vi "Tigella_Main.vi"() -> ()   [LabVIEW 2024]
uses:
  PS3 Control V8.6/Controls/PS3 Controls.ctl
  <vilib>/Instr/_visa.llb/VISA Set IO Buffer Mask.ctl
  <vilib>/Instr/_visa.llb/VISA Configure Serial Port (Instr).vi
panel:
  out "MOF_Motor2":u8=3
  out "MOF_Motor1":u8=2
  out "read buffer":string
  out "return count":u32
  in  "VISA resource name out":refnum<visa-resource-name>
  in  "parity (0:none)":enum16{"None", "Odd", "Even", "Mark", "Space"}(ring)
  in  "data bits (8)":u16=8 min=5 max=8 step=1
  in  "baud rate (9600)":u32=115200
  out "M2_I_Adsorbed":i64
  out "M1_I_Adsorbed":i64
  out "Warning_M2":bool=TRUE
  out "Warning_M1":bool=TRUE
  out "Error_M2":bool=TRUE
  out "Error_M1":bool=TRUE
  out "STM _WIFIConnected":bool
  in  "Tab Control":T1(tab)
  out "Listbox_Motors_errors":i32(listbox)
  in  "Homing_M1":bool
  in  "velocity_profileM1":bool
  in  "position_profile_M1":bool
  out "Actual_Modality_M1":string
  in  "Start_Remote_Node_M1":bool
  in  "Stop_Remote_Node_M1":bool
  in  "Reset_Node_M1":bool
  in  "Reset_Communication_M1":bool
  in  "Enter_Pre_Operational_M1":bool
  out "NMT_State_M1":string
  in  "Shutdown_M1":bool
  out "Driver_State_M1":string
  in  "Disable_voltage_M1":bool
  in  "Switch_On_M1":bool
  in  "Disable_operation_M1":bool
  in  "Enable_Operation_M1":bool
  in  "Fault_Reset_M1":bool
  in  "Quick_Stop_M1":bool
  in  "Quick_Stop_M2":bool
  in  "Fault_Reset_M2":bool
  in  "Enable_Operation_M2":bool
  in  "Disable_operation_M2":bool
  in  "Switch_On_M2":bool
  in  "Disable_voltage_M2":bool
  out "Driver_State_M2":string
  in  "Shutdown_M2":bool
  out "NMT_State_M2":string
  in  "Enter_Pre_Operational_M2":bool
  in  "Reset_Communication_M2":bool
  in  "Reset_Node_M2":bool
  in  "Stop_Remote_Node_M2":bool
  in  "Start_Remote_Node_M2":bool
  out "Actual_Modality_M2":string
  in  "position_profile_M2":bool
  in  "velocity_profileM2":bool
  in  "Homing_M2":bool
  out "Listbox_Motors_errors 2":i32(listbox)
  in  "Halt_M2":bool
  out "M2_Velocity":i64
  out "M2_Position":i64
  in  "Change_set_immediately_M2":bool=TRUE
  in  "ABS/REL_M2":bool=TRUE
  in  "Target_Position_M2":i32
  in  "Target_speed_M2":i32
  in  "GO_TO_M2":bool
  out "M2_Following/homing error":bool=TRUE
  out "M2_Setpoint acknowledge/Homing attained":bool=TRUE
  out "M2_target_reached":bool=TRUE
  out "Saved_position_negative_M2":i64
  out "Saved_position_positive_M2":i64
  out "Motor2_FULL_Operational":bool=TRUE
  in  "Halt_M1":bool
  out "End-Stop_sensor":bool=TRUE
  out "Homing_Sensor":bool=TRUE
  out "M1_Velocity":i64
  out "M1_Position":i64
  in  "Change_set_immediately_M1":bool=TRUE
  in  "ABS/REL_M1":bool=TRUE
  in  "Target_Position_M1":i32
  in  "Target_speed_M1":i32
  in  "GO_TO_M1":bool
  out "M1_Following/homing error":bool=TRUE
  out "M1_Setpoint acknowledge/Homing attained":bool=TRUE
  out "M1_Internal_limit_\nactive":bool=TRUE
  out "M1_target_reached":bool=TRUE
  out "Saved_position_negative_M1":i64
  out "Saved_position_positive_M1":i64
  out "Motor1_FULL_Operational":bool=TRUE
  in  "Open_CAM":bool
  out "Controller_ERROR_STATUS":errorcluster
  out "PS3/4_controller_status":bool
  in  "Connect_PS3/4_controller":bool
  out "PS3 Controls":T2 {"Left Analogue Stick X" scale=-32768.0..32768.0; "Left Analogue Stick Y" scale=32768.0..-32768.0; "Right Analogue Stick X" scale=-32768.0..32768.0; "Right Analogue Stick Y" scale=32768.0..-32768.0; "X Rotation" scale=-32768.0..32768.0; "Y Rotation" scale=-32768.0..32768.0; "L2 Pressure" scale=0.0..32768.0; "Numeric" format="%d°"}
  in  "ID_Motor2":u8=3
  in  "ID_Motor1":u8=2
  out "Position_traction":i64
  out "Position_steering":i64
  out "Velocity_Traction":i64
  out "Velocity_steering":i64
  in  "SET_nodes":bool
  in  "DISCONNECT":bool
  in  "CONNECT":bool
  in  "kind-connection":bool=TRUE caption="Boolean"
  in  "exit all":bool
  out "STM _SeialConnected":bool
  out "error out":errorcluster
  # "ID"
  # "Motor1-Steering"
  # "Velocity (rad/s)"
  # "Position (INC)"
  # "Position(INC)"
  # "Velocity(rad/s)"
  # "Motor2-Traction"
  # "Motor1-Steering"
  # "Motor2-Traction"
  # "mm/s"
  # "mm/s"
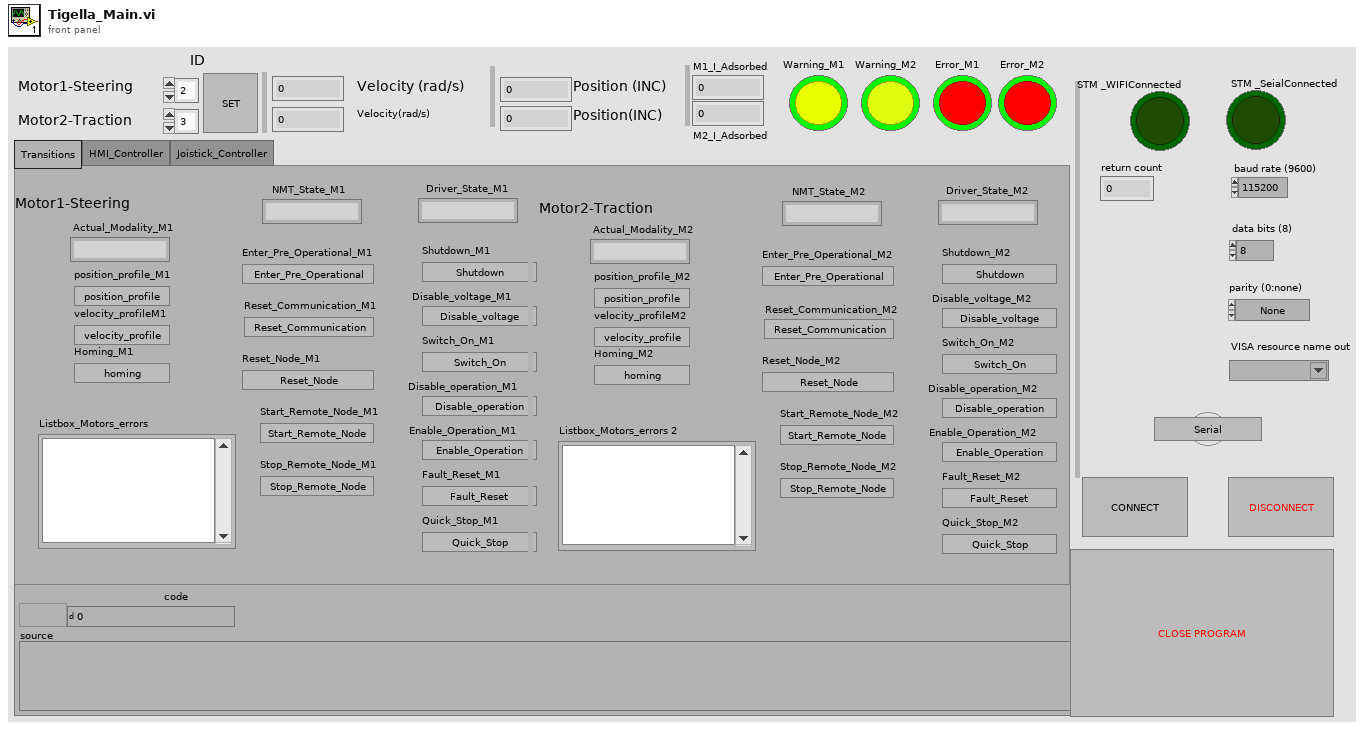
[diagram p1: front panel]
types:
  T1 = enum32{"Transitions", "HMI_Controller", "Joistick_Controller"}
  T2 = typedef "PS3 Controls.ctl" = cluster{"Left Analogue Stick X":i32, "Left Analogue Stick Y":i32, "Right Analogue Stick X":i32, "Right Analogue Stick Y":i32, "Y Rotation":i32, "X Rotation":i32, "L2 Pressure":i32, "R2 Pressure":i32, "Triangle":bool, "Circle":bool, "X":bool, "Square":bool, "L1":bool, "R1":bool, "L2":bool, "R2":bool, "L3":bool, "R3":bool, "Select":bool, "Start":bool, "PS Button":bool, "Numeric":i32}
  T3 = typedef "VISA Set IO Buffer Mask.ctl" = u16
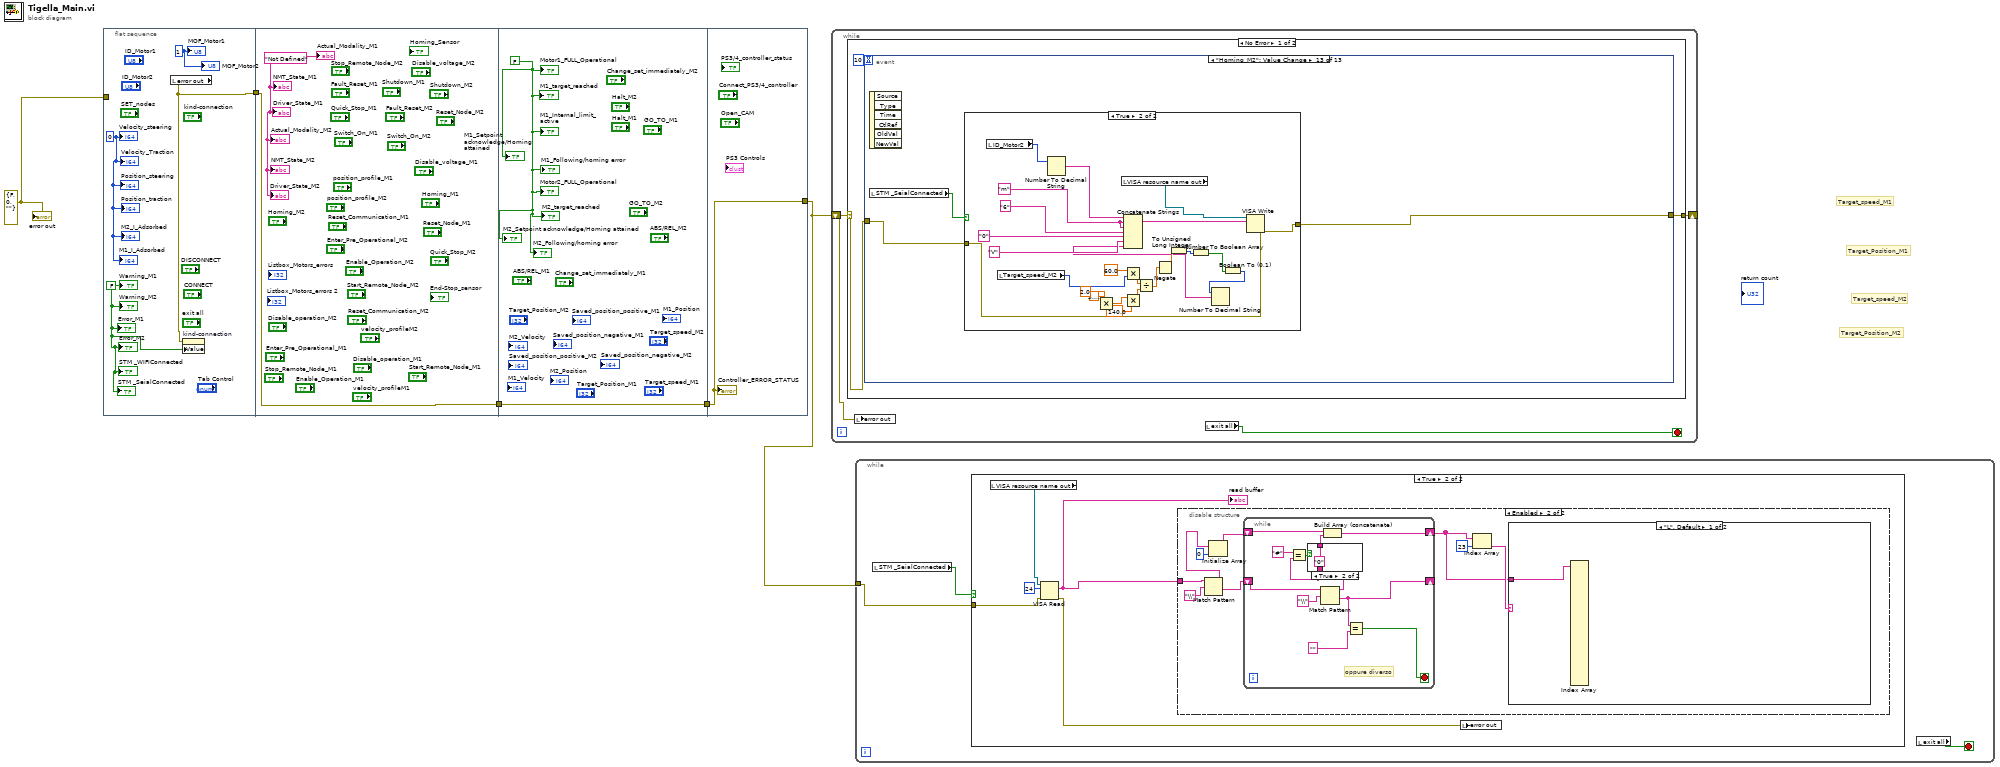
[diagram p0: block diagram]
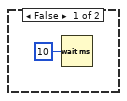
[diagram p2: hidden frame]
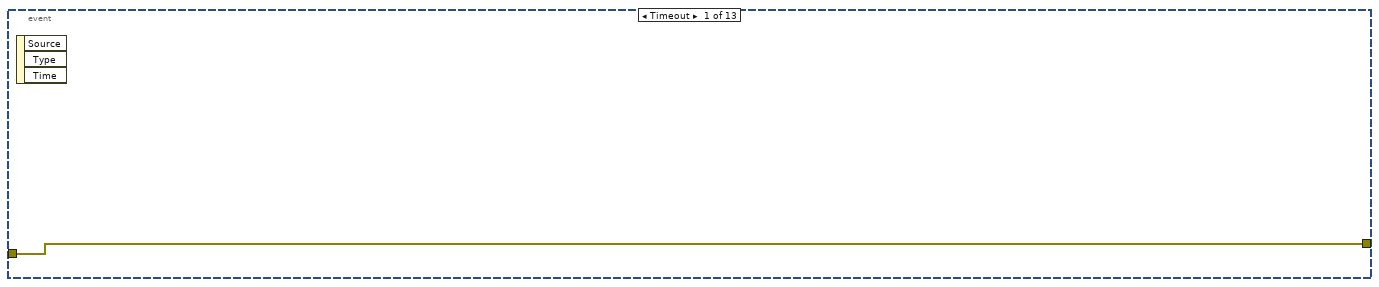
[diagram p6: hidden frame]
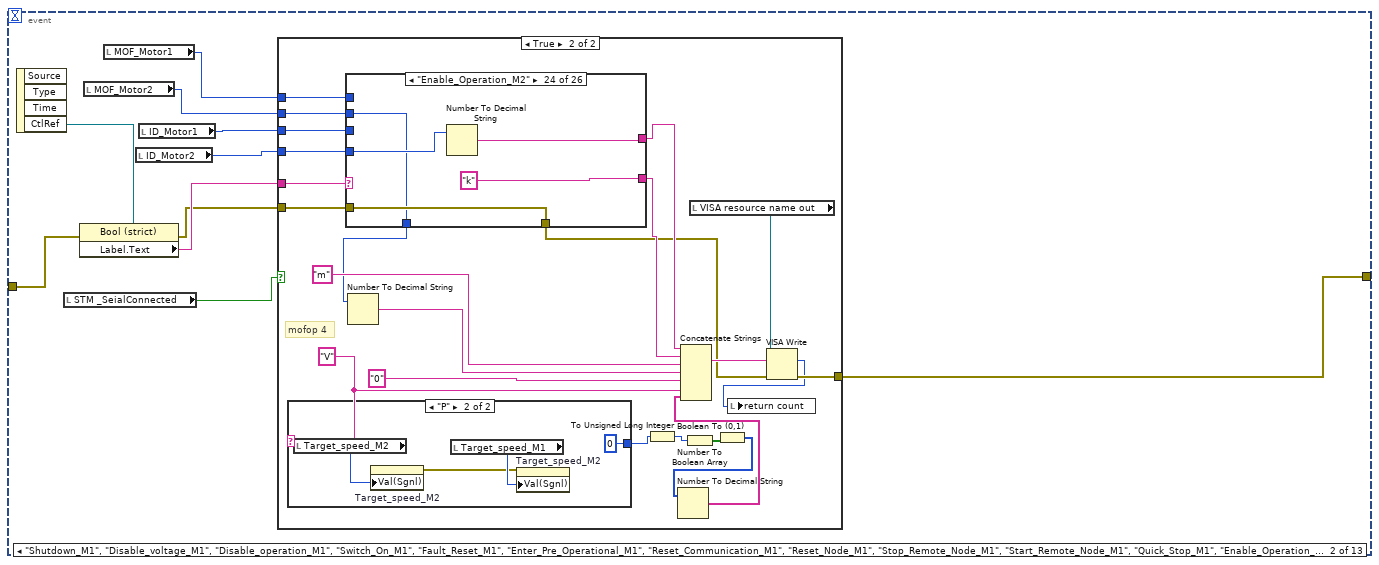
[diagram p7: hidden frame]
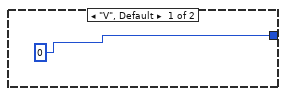
[diagram p9: hidden frame]
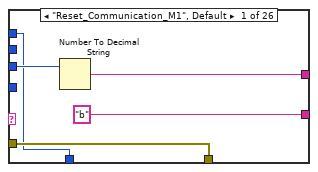
[diagram p10: hidden frame]
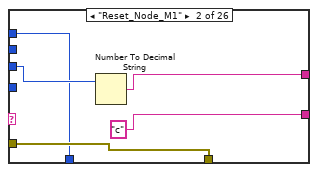
[diagram p11: hidden frame]
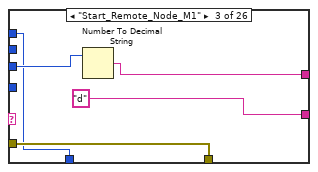
[diagram p12: hidden frame]
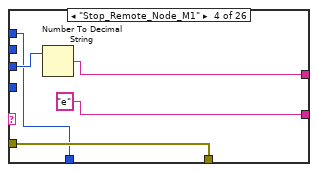
[diagram p13: hidden frame]
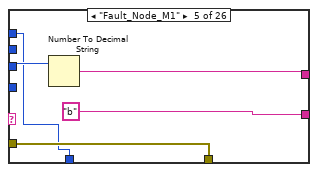
[diagram p14: hidden frame]
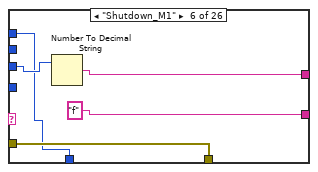
[diagram p15: hidden frame]
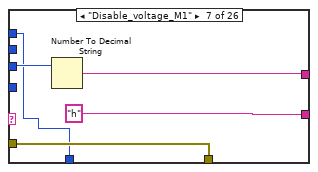
[diagram p16: hidden frame]
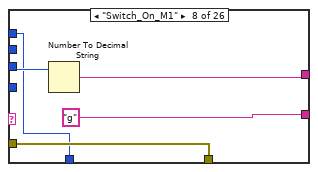
[diagram p17: hidden frame]
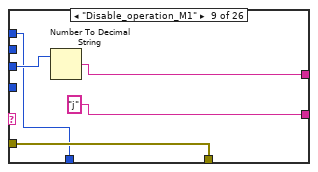
[diagram p18: hidden frame]
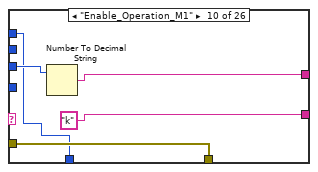
[diagram p19: hidden frame]
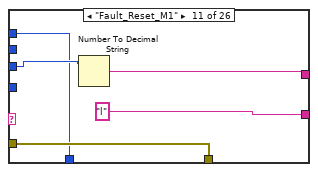
[diagram p20: hidden frame]
diagram:
  w4 = errorcluster {"status"=FALSE, "code"=0, "source"=""} ("error out")
  # "Target_Position_M2"
  # "Target_speed_M2"
  # "Target_Position_M1"
  # "Target_speed_M1"
  n1 = flat-sequence {
    tunnel: [w8] -> w5
    tunnel: w4 -> [_]
    tunnel: w5 -> [w10]
    tunnel: [w10] -> w3
    tunnel: w3 -> [w12]
    tunnel: [w12] -> w2
    tunnel: w2 -> [w14]
    tunnel: [w14] -> w1
    frame #0 {
      w6 = u8 1 ("MOF_Motor1")
      w9 = FALSE ("Warning_M1")
      w7 = i64 0 ("Velocity_steering")
      n2 = local read "error out"() -> (w8:errorcluster)
      n3 = property on="kind-connection" class="Bool (strict)"(error in=w8, "Value"=w9) -> ()  [unwired: 1 in, 2 out]
      "Velocity_steering" <- w7
      "Velocity_Traction" <- w7
      "Position_traction" <- w7
      "Position_steering" <- w7
      "M2_I_Adsorbed" <- w7
      "Warning_M1" <- w9
      "Warning_M2" <- w9
      "Error_M1" <- w9
      "Error_M2" <- w9
      "STM _WIFIConnected" <- w9
      "STM _SeialConnected" <- w9
      "M1_I_Adsorbed" <- w7
      "MOF_Motor1" <- w6
      "MOF_Motor2" <- w6
    }
    frame #1 {
      w11 = "Not Defined" ("Actual_Modality_M1")
      "Actual_Modality_M1" <- w11
      "NMT_State_M1" <- w11
      "Driver_State_M1" <- w11
      "Actual_Modality_M2" <- w11
      "NMT_State_M2" <- w11
      "Driver_State_M2" <- w11
    }
    frame #2 {
      w13 = FALSE ("Motor1_FULL_Operational")
      "Motor1_FULL_Operational" <- w13
      "M1_target_reached" <- w13
      "M1_Internal_limit_\nactive" <- w13
      "M1_Setpoint acknowledge/Homing attained" <- w13
      "M1_Following/homing error" <- w13
      "Motor2_FULL_Operational" <- w13
      "M2_target_reached" <- w13
      "M2_Setpoint acknowledge/Homing attained" <- w13
      "M2_Following/homing error" <- w13
    }
    frame #3 {
      "Controller_ERROR_STATUS" <- w14
    }
  }
  n4 = while {
    shift-right: [w17] -> _
    shift-left: w1 -> [w16]
    stop <- w15 stop-if-true
    n5 = case shown="No Error" w16 {
      selector: w16 -> [w19 w581]
      tunnel: [w18 errorcluster {"status"=FALSE, "code"=0, "source"=""} ("error in (no error)")] -> w17
      frame No Error {
        n6 = event shown="[12] \"Homing_M2\": Value Change" {
          selector: _ -> [_ _ _ _ _ _ _ _ _ _ _ _ _]
          dyn-events: _ -> [_ _ _ _ _ _ _ _ _ _ _ _ _]
          timeout: 10 -> [_ _ _ _ _ _ _ _ _ _ _ _ _]
          tunnel: w19 -> [w21 w29 w199 w271 w396 w411 w427 w429 w458 w478 w507 w527 w555]
          tunnel: [w21 w25 w196 w265 w396 w403 w426 w430 w459 w477 w505 w526 w554] -> w18
          event Timeout {
            n7 = event-data() -> ()  [unwired: 1 in, 3 out]
          }
          event "Shutdown_M1", "Disable_voltage_M1", "Disable_operation_M1", "Switch_On_M1", "Fault_Reset_M1", "Enter_Pre_Operational_M1", "Reset_Communication_M1", "Reset_Node_M1", "Stop_Remote_Node_M1", "Start_Remote_Node_M1", "Quick_Stop_M1", "Enable_Operation_M2", "Disable_operation_M2", "Switch_On_M2", "Disable_voltage_M2", "Shutdown_M2", "Enter_Pre_Operational_M2", "Reset_Communication_M2", "Reset_Node_M2", "Stop_Remote_Node_M2", "Start_Remote_Node_M2", "Quick_Stop_M2", "Enable_Operation_M1": Mouse Down; "Enable_Operation_M1": Key Down {
            n8 = event-data() -> ("CtlRef"=w31:refnum<vi>)  [unwired: 1 in, 3 out]
            n9 = local read "STM _SeialConnected"() -> (w24:bool)
            n10 = property on="Property Node" class="Bool (strict)"(reference=w31, error in=w29) -> (error out=w28:errorcluster, "Label.Text"=w30:string)  [unwired: 1 out]
            n11 = local read "MOF_Motor2"() -> (w22:u8)
            n12 = local read "MOF_Motor1"() -> (w23:u8)
            n13 = local read "ID_Motor2"() -> (w26:u8)
            n14 = local read "ID_Motor1"() -> (w27:u8)
            n15 = case shown="True" w24 {
              tunnel: w30 -> [_ w55]
              tunnel: w28 -> [w32 w54]
              tunnel: w27 -> [_ w42]
              tunnel: w26 -> [_ w41]
              tunnel: [w32 w39] -> w25
              tunnel: w23 -> [_ w35]
              tunnel: w22 -> [_ w34]
              frame False {
              }
              frame True {
                w47 = "V" ("comand")
                # "mofop 4"
                n16 = case shown="\"P\"" w47 {
                  tunnel: [u8 0 ("Touch_probe") u8 0 ("Touch_probe")] -> w50
                  frame "V", Default {
                  }
                  frame "P" {
                    n17 = local read "Target_speed_M2"() -> (w60:i32)
                    n18 = property on="Target_speed_M2" class="DigNum (strict)"("Val(Sgnl)"=w60) -> (error out=w58:errorcluster)  [unwired: 2 in, 1 out]
                    n19 = local read "Target_speed_M1"() -> (w59:i32)
                    n20 = property on="Target_speed_M2" class="DigNum (strict)"(error in=w58, "Val(Sgnl)"=w59) -> ()  [unwired: 1 in, 2 out]
                  }
                }
                n21 = case shown="\"Enable_Operation_M2\"" w55 {
                  tunnel: w54 -> [w62 w67 w72 w77 w82 w87 w92 w97 w102 w107 w112 w117 w122 w127 w132 w137 w142 w147 w152 w157 w162 w167 w172 w177 w182 w187]
                  tunnel: [w65 w70 w75 w80 w85 w90 w95 w100 w105 w110 w115 w120 w125 w130 w135 w140 w145 w150 w155 w160 w165 w170 w175 w180 w185 w190] -> w44
                  tunnel: ["b" ("transitions") "c" ("transitions") "d" ("transitions") "e" ("transitions") "b" ("transitions") "f" ("transitions") "h" ("transitions") "g" ("transitions") "j" ("transitions") "k" ("transitions") "l" ("transitions") "a" ("transitions") "i" ("transitions") "a" ("transitions") "b" ("transitions") "c" ("transitions") "d" ("transitions") "e" ("transitions") "b" ("transitions") "f" ("transitions") "h" ("transitions") "g" ("transitions") "j" ("transitions") "k" ("transitions") "l" ("transitions") "i" ("transitions")] -> w43
                  tunnel: w42 -> [w63 w69 w74 w79 w84 w89 w94 w99 w104 w109 w114 w119 w124 _ _ _ _ _ _ _ _ _ _ _ _ _]
                  tunnel: w41 -> [_ _ _ _ _ _ _ _ _ _ _ _ _ w129 w134 w139 w144 w149 w154 w159 w164 w169 w174 w179 w184 w189]
                  tunnel: [w62 w67 w72 w77 w82 w87 w92 w97 w102 w107 w112 w117 w122 w127 w132 w137 w142 w147 w152 w157 w162 w167 w172 w177 w182 w187] -> w40
                  tunnel: w35 -> [w61 w66 w71 w76 w81 w86 w91 w96 w101 w106 w111 w116 w121 _ _ _ _ _ _ _ _ _ _ _ _ _]
                  tunnel: w34 -> [_ _ _ _ _ _ _ _ _ _ _ _ _ w126 w131 w136 w141 w146 w151 w156 w161 w166 w171 w176 w181 w186]
                  tunnel: [w61 w66 w71 w76 w81 w86 w91 w96 w101 w106 w111 w116 w121 w126 w131 w136 w141 w146 w151 w156 w161 w166 w171 w176 w181 w186] -> w33
                  frame "Reset_Communication_M1", Default {
                    n22 = Number To Decimal String(number=w63) -> (decimal integer string=w65:string)  [unwired: 1 in]
                  }
                  frame "Reset_Node_M1" {
                    n23 = Number To Decimal String(number=w69) -> (decimal integer string=w70:string)  [unwired: 1 in]
                  }
                  frame "Start_Remote_Node_M1" {
                    n24 = Number To Decimal String(number=w74) -> (decimal integer string=w75:string)  [unwired: 1 in]
                  }
                  frame "Stop_Remote_Node_M1" {
                    n25 = Number To Decimal String(number=w79) -> (decimal integer string=w80:string)  [unwired: 1 in]
                  }
                  frame "Fault_Node_M1" {
                    n26 = Number To Decimal String(number=w84) -> (decimal integer string=w85:string)  [unwired: 1 in]
                  }
                  frame "Shutdown_M1" {
                    n27 = Number To Decimal String(number=w89) -> (decimal integer string=w90:string)  [unwired: 1 in]
                  }
                  frame "Disable_voltage_M1" {
                    n28 = Number To Decimal String(number=w94) -> (decimal integer string=w95:string)  [unwired: 1 in]
                  }
                  frame "Switch_On_M1" {
                    n29 = Number To Decimal String(number=w99) -> (decimal integer string=w100:string)  [unwired: 1 in]
                  }
                  frame "Disable_operation_M1" {
                    n30 = Number To Decimal String(number=w104) -> (decimal integer string=w105:string)  [unwired: 1 in]
                  }
                  frame "Enable_Operation_M1" {
                    n31 = Number To Decimal String(number=w109) -> (decimal integer string=w110:string)  [unwired: 1 in]
                  }
                  frame "Fault_Reset_M1" {
                    n32 = Number To Decimal String(number=w114) -> (decimal integer string=w115:string)  [unwired: 1 in]
                  }
                  frame "Enter_Pre_Operational_M1" {
                    n33 = Number To Decimal String(number=w119) -> (decimal integer string=w120:string)  [unwired: 1 in]
                  }
                  frame "Quick_Stop_M1" {
                    n34 = Number To Decimal String(number=w124) -> (decimal integer string=w125:string)  [unwired: 1 in]
                  }
                  frame "Enter_Pre_Operational_M2" {
                    n35 = Number To Decimal String(number=w129) -> (decimal integer string=w130:string)  [unwired: 1 in]
                  }
                  frame "Reset_Communication_M2" {
                    n36 = Number To Decimal String(number=w134) -> (decimal integer string=w135:string)  [unwired: 1 in]
                  }
                  frame "Reset_Node_M2" {
                    n37 = Number To Decimal String(number=w139) -> (decimal integer string=w140:string)  [unwired: 1 in]
                  }
                  frame "Start_Remote_Node_M2" {
                    n38 = Number To Decimal String(number=w144) -> (decimal integer string=w145:string)  [unwired: 1 in]
                  }
                  frame "Stop_Remote_Node_M2" {
                    n39 = Number To Decimal String(number=w149) -> (decimal integer string=w150:string)  [unwired: 1 in]
                  }
                  frame "Fault_Node_M2" {
                    n40 = Number To Decimal String(number=w154) -> (decimal integer string=w155:string)  [unwired: 1 in]
                  }
                  frame "Shutdown_M2" {
                    n41 = Number To Decimal String(number=w159) -> (decimal integer string=w160:string)  [unwired: 1 in]
                  }
                  frame "Disable_voltage_M2" {
                    n42 = Number To Decimal String(number=w164) -> (decimal integer string=w165:string)  [unwired: 1 in]
                  }
                  frame "Switch_On_M2" {
                    n43 = Number To Decimal String(number=w169) -> (decimal integer string=w170:string)  [unwired: 1 in]
                  }
                  frame "Disable_operation_M2" {
                    n44 = Number To Decimal String(number=w174) -> (decimal integer string=w175:string)  [unwired: 1 in]
                  }
                  frame "Enable_Operation_M2" {
                    n45 = Number To Decimal String(number=w179) -> (decimal integer string=w180:string)  [unwired: 1 in]
                  }
                  frame "Fault_Reset_M2" {
                    n46 = Number To Decimal String(number=w184) -> (decimal integer string=w185:string)  [unwired: 1 in]
                  }
                  frame "Quick_Stop_M2" {
                    n47 = Number To Decimal String(number=w189) -> (decimal integer string=w190:string)  [unwired: 1 in]
                  }
                }
                n48 = Number To Decimal String(number=w33) -> (decimal integer string=w48:string)  [unwired: 1 in]
                n49 = To Unsigned Long Integer(number=w50) -> (unsigned 32bit integer=w52:u32)
                n50 = Number To Boolean Array(number=w52) -> (Boolean array=w51:bool[])
                n51 = local read "VISA resource name out"() -> (w38:refnum<visa-resource-name>)
                n52 = Boolean To (0,1)(Boolean=w51) -> (0, 1=w49:i16[])
                n53 = Number To Decimal String(number=w49) -> (decimal integer string=w46:string[])  [unwired: 1 in]
                n54 = Concatenate Strings(w44, w43, "m" ("Emergency_comand"), w48, "0" ("string"), w47, w46) -> (w45:string)
                n55 = VISA Write(VISA resource name=w38, write buffer=w45, error in (no error)=w40) -> (return count=w36:u32, error out=w39:errorcluster)  [unwired: 1 out]
                n56 = local write "return count"(w36) -> ()
              }
            }
          }
          event "Target_speed_M1", "Target_Position_M1", "Target_speed_M2", "Target_Position_M2": Value Change {
            n57 = event-data() -> ("CtlRef"=w200:refnum<vi>)  [unwired: 1 in, 5 out]
            n58 = local read "STM _SeialConnected"() -> (w198:bool)
            n59 = property on="Property Node" class="DigNum (strict)"(reference=w200, error in=w199) -> (error out=w197:errorcluster, "Label.Text"=w193:string)  [unwired: 1 out]
            n60 = local read "MOF_Motor2"() -> (w191:u8)
            n61 = local read "MOF_Motor1"() -> (w192:u8)
            n62 = local read "ID_Motor2"() -> (w194:u8)
            n63 = local read "ID_Motor1"() -> (w195:u8)
            n64 = case shown="True" w198 {
              tunnel: w197 -> [w201 w210]
              tunnel: [w201 w209] -> w196
              tunnel: w195 -> [_ w223]
              tunnel: w194 -> [_ w222]
              tunnel: w193 -> [_ w221]
              tunnel: w192 -> [_ w207]
              tunnel: w191 -> [_ w206]
              frame False {
              }
              frame True {
                w218 = "m" ("transitions")
                n65 = case shown="\"Target_speed_M2\"" w221 {
                  tunnel: [w237 w251 w256 w261] -> w219
                  tunnel: ["V" ("transitions") "V" ("transitions") "P" ("transitions") "P" ("transitions")] -> w216
                  tunnel: w222 -> [_ w250 _ w258]
                  tunnel: w223 -> [w236 _ w254 _]
                  tunnel: [w234 w248 w253 w259] -> w202
                  tunnel: w207 -> [w233 _ w252 _]
                  tunnel: w206 -> [_ w247 _ w257]
                  tunnel: [w233 w247 w252 w257] -> w205
                  frame "Target_speed_M1", Default {
                    n66 = local read "Target_speed_M1"() -> (w224:i32)
                    n67 = Number To Decimal String(number=w236) -> (decimal integer string=w237:string)  [unwired: 1 in]
                    n68 = Multiply(x=2.0, y=3.141592653589793) -> (x*y=w228:dbl)
                    n69 = Multiply(x=60.0, y=w224) -> (x*y=w231:dbl)
                    n70 = Multiply(x=w228, y=140.0 ("x")) -> (x*y=w226:dbl)
                    n71 = Divide(x=w231, y=w226) -> (x/y=w225:dbl)
                    n72 = Negate(x=w225) -> (-x=w234:dbl)
                  }
                  frame "Target_speed_M2" {
                    n73 = local read "Target_speed_M2"() -> (w238:i32)
                    n74 = Number To Decimal String(number=w250) -> (decimal integer string=w251:string)  [unwired: 1 in]
                    n75 = Multiply(x=2.0, y=3.141592653589793) -> (x*y=w241:dbl)
                    n76 = Multiply(x=60.0, y=w238) -> (x*y=w244:dbl)
                    n77 = Multiply(x=w241, y=140.0 ("x")) -> (x*y=w239:dbl)
                    n78 = Divide(x=w244, y=w239) -> (x/y=w245:dbl)
                    n79 = Negate(x=w245) -> (-x=w248:dbl)
                  }
                  frame "Target_Position_M1" {
                    n80 = Number To Decimal String(number=w254) -> (decimal integer string=w256:string)  [unwired: 1 in]
                    n81 = local read "Target_Position_M1"() -> (w253:i32)
                  }
                  frame "Target_Position_M2" {
                    n82 = Number To Decimal String(number=w258) -> (decimal integer string=w261:string)  [unwired: 1 in]
                    n83 = local read "Target_Position_M2"() -> (w259:i32)
                  }
                }
                n84 = Number To Decimal String(number=w205) -> (decimal integer string=w204:string)  [unwired: 1 in]
                n85 = local read "VISA resource name out"() -> (w211:refnum<visa-resource-name>)
                n86 = To Long Integer(number=w202) -> (32bit integer=w203:i32)
                n87 = To Unsigned Long Integer(number=w203) -> (unsigned 32bit integer=w215:u32)
                n88 = Number To Boolean Array(number=w215) -> (Boolean array=w214:bool[])
                n89 = Boolean To (0,1)(Boolean=w214) -> (0, 1=w213:i16[])
                n90 = Number To Decimal String(number=w213) -> (decimal integer string=w212:string[])  [unwired: 1 in]
                n91 = Concatenate Strings(w219, w218, w218, w204, "0" ("transitions"), w216, w212) -> (w220:string)
                n92 = VISA Write(VISA resource name=w211, write buffer=w220, error in (no error)=w210) -> (return count=w208:u32, error out=w209:errorcluster)  [unwired: 1 out]
                n93 = local write "return count"(w208) -> ()
              }
            }
          }
          event "Halt_M1", "Halt_M2", "Change_set_immediately_M1", "Change_set_immediately_M2", "ABS/REL_M1", "ABS/REL_M2", "GO_TO_M1", "GO_TO_M2": Value Change {
            n94 = event-data() -> ("CtlRef"=w272:refnum<vi>, "NewVal"=w264:bool)  [unwired: 1 in, 4 out]
            n95 = local read "STM _SeialConnected"() -> (w269:bool)
            n96 = local read "ID_Motor2"() -> (w267:u8)
            n97 = local read "ID_Motor1"() -> (w268:u8)
            n98 = local read "MOF_Motor1"() -> (w263:u8)
            n99 = local read "MOF_Motor2"() -> (w262:u8)
            n100 = property on="Property Node" class="Bool"(reference=w272, error in=w271) -> (error out=w266:errorcluster, "Label.Text"=w270:string)  [unwired: 1 out]
            n101 = case shown="True" w269 {
              tunnel: w270 -> [_ w315]
              tunnel: w268 -> [_ w314]
              tunnel: w267 -> [_ w313]
              tunnel: w266 -> [w273 w312]
              tunnel: [w273 w299] -> w265
              tunnel: w264 -> [_ w301]
              tunnel: w263 -> [_ w296]
              tunnel: w262 -> [_ w295]
              frame False {
              }
              frame True {
                n102 = local read "Target_speed_M1"() -> (w285:i32)
                n103 = local read "Target_speed_M2"() -> (w277:i32)
                n104 = Multiply(x=2.0, y=3.141592653589793) -> (x*y=w288:dbl)
                n105 = Multiply(x=60.0, y=w285) -> (x*y=w291:dbl)
                n106 = Multiply(x=w288, y=140.0 ("x")) -> (x*y=w286:dbl)
                n107 = Divide(x=w291, y=w286) -> (x/y=w276:dbl)
                n108 = Multiply(x=2.0, y=3.141592653589793) -> (x*y=w280:dbl)
                n109 = Multiply(x=60.0, y=w277) -> (x*y=w283:dbl)
                n110 = Multiply(x=w280, y=140.0 ("x")) -> (x*y=w278:dbl)
                n111 = Divide(x=w283, y=w278) -> (x/y=w275:dbl)
                n112 = case shown="\"GO_TO_M1\"" w315 {
                  tunnel: w312 -> [w321 w331 w339 w350 w362 w372 w381 w392]
                  tunnel: [w323 w333 w342 w352 w363 w373 w383 w393] -> w304
                  tunnel: [w319 w329 w340 w349 w360 w369 w379 w390] -> w302
                  tunnel: w314 -> [w322 w332 w343 _ _ _ w382 _]
                  tunnel: [w321 w331 w339 w350 w362 w372 w381 w392] -> w300
                  tunnel: w313 -> [_ _ _ w353 w361 w371 _ w391]
                  tunnel: w301 -> [w320 w330 w341 w351 w359 w370 w380 w389]
                  tunnel: w296 -> [w318 w328 w338 _ _ _ w378 _]
                  tunnel: w295 -> [_ _ _ w348 w358 w368 _ w388]
                  tunnel: [w318 w328 w338 w348 w358 w368 w378 w388] -> w294
                  tunnel: w276 -> [w317 w327 w337 _ _ _ w377 _]
                  tunnel: w275 -> [_ _ _ w347 w357 w367 _ w387]
                  tunnel: [w316 w326 w336 w346 w356 w366 w376 w386] -> w274
                  frame "ABS/REL_M1", Default {
                    n113 = To Long Integer(number=w317) -> (32bit integer=w316:i32)
                    n114 = Number To Decimal String(number=w322) -> (decimal integer string=w323:string)  [unwired: 1 in]
                    n115 = case shown="False" w320 {
                      tunnel: ["6" ("transitions") "7" ("transitions")] -> w319
                      frame False {
                      }
                      frame True {
                      }
                    }
                  }
                  frame "Change_set_immediately_M1" {
                    n116 = To Long Integer(number=w327) -> (32bit integer=w326:i32)
                    n117 = Number To Decimal String(number=w332) -> (decimal integer string=w333:string)  [unwired: 1 in]
                    n118 = case shown="True" w330 {
                      tunnel: ["4" ("transitions") "5" ("transitions")] -> w329
                      frame False {
                      }
                      frame True {
                      }
                    }
                  }
                  frame "GO_TO_M1" {
                    n119 = To Long Integer(number=w337) -> (32bit integer=w336:i32)
                    n120 = Number To Decimal String(number=w343) -> (decimal integer string=w342:string)  [unwired: 1 in]
                    n121 = case shown="True" w341 {
                      tunnel: ["2" ("transitions") "3" ("transitions")] -> w340
                      frame False {
                      }
                      frame True {
                      }
                    }
                  }
                  frame "GO_TO_M2" {
                    n122 = To Long Integer(number=w347) -> (32bit integer=w346:i32)
                    n123 = Number To Decimal String(number=w353) -> (decimal integer string=w352:string)  [unwired: 1 in]
                    n124 = case shown="False" w351 {
                      tunnel: ["2" ("transitions") "3" ("transitions")] -> w349
                      frame False {
                      }
                      frame True {
                      }
                    }
                  }
                  frame "ABS/REL_M2" {
                    n125 = To Long Integer(number=w357) -> (32bit integer=w356:i32)
                    n126 = Number To Decimal String(number=w361) -> (decimal integer string=w363:string)  [unwired: 1 in]
                    n127 = case shown="True" w359 {
                      tunnel: ["6" ("transitions") "7" ("transitions")] -> w360
                      frame False {
                      }
                      frame True {
                      }
                    }
                  }
                  frame "Change_set_immediately_M2" {
                    n128 = To Long Integer(number=w367) -> (32bit integer=w366:i32)
                    n129 = Number To Decimal String(number=w371) -> (decimal integer string=w373:string)  [unwired: 1 in]
                    n130 = case shown="False" w370 {
                      tunnel: ["4" ("transitions") "5" ("transitions")] -> w369
                      frame False {
                      }
                      frame True {
                      }
                    }
                  }
                  frame "Halt_M1" {
                    n131 = To Long Integer(number=w377) -> (32bit integer=w376:i32)
                    n132 = Number To Decimal String(number=w382) -> (decimal integer string=w383:string)  [unwired: 1 in]
                    n133 = case shown="False" w380 {
                      tunnel: ["0" ("transitions") "1" ("transitions")] -> w379
                      frame False {
                      }
                      frame True {
                      }
                    }
                  }
                  frame "Halt_M2" {
                    n134 = To Long Integer(number=w387) -> (32bit integer=w386:i32)
                    n135 = Number To Decimal String(number=w391) -> (decimal integer string=w393:string)  [unwired: 1 in]
                    n136 = case shown="False" w389 {
                      tunnel: ["0" ("transitions") "1" ("transitions")] -> w390
                      frame False {
                      }
                      frame True {
                      }
                    }
                  }
                }
                n137 = To Unsigned Long Integer(number=w274) -> (unsigned 32bit integer=w311:u32)
                n138 = Number To Boolean Array(number=w311) -> (Boolean array=w310:bool[])
                n139 = Boolean To (0,1)(Boolean=w310) -> (0, 1=w309:i16[])
                n140 = Number To Decimal String(number=w294) -> (decimal integer string=w308:string)  [unwired: 1 in]
                n141 = Number To Decimal String(number=w309) -> (decimal integer string=w306:string[])  [unwired: 1 in]
                n142 = local read "VISA resource name out"() -> (w298:refnum<visa-resource-name>)
                n143 = Concatenate Strings(w304, "m" ("Emergency_comand"), w302, w308, "0" ("comand"), "V" ("comand"), w306) -> (w305:string)
                n144 = VISA Write(VISA resource name=w298, write buffer=w305, error in (no error)=w300) -> (return count=w297:u32, error out=w299:errorcluster)  [unwired: 1 out]
                n145 = local write "return count"(w297) -> ()
              }
            }
          }
          event "exit all": Mouse Down {
            n146 = event-data() -> ()  [unwired: 1 in, 8 out]
            n147 = Wait (ms)(milliseconds to wait=u32 10) -> ()  [unwired: 1 out]
          }
          event "CONNECT": Mouse Down {
            w401 = T3 16 items=["I/O Receive Buffer"=16, "I/O Transmit Buffer"=32, "I/O Receive and Transmit Buffer"=48] ("Mask")
            w408 = T3 32 items=["I/O Receive Buffer"=16, "I/O Transmit Buffer"=32, "I/O Receive and Transmit Buffer"=48] ("Mask")
            w412 = u16 0 items=["None", "XON/XOFF", "RTS/CTS", "XON/XOFF & RTS/CTS", "DTR/DSR", "XON/XOFF & DTR/DSR"] ("flow control (0:none)")
            w413 = u16 10 items=["1.0"=10, "1.5"=15, "2.0"=20] ("stop bits (10: 1 bit)")
            n148 = event-data() -> ()  [unwired: 1 in, 8 out]
            n149 = call-poly "VISA Configure Serial Port"("VISA resource name"="VISA resource name out", "termination char\n(0xA = '\\n' = LF)"=u8 10 ("termination char\n(0xA = '\\n' = LF)"), "Enable Termination\nChar (T)"=TRUE ("Enable Termination\nChar (T)"), "baud rate (9600)"="baud rate (9600)", "data bits (8)"="data bits (8)", "parity (0:none)"="parity (0:none)", "error in (no error)"=w411, "stop bits (10: 1 bit)"=w413, "flow control (0:none)"=w412) -> ("VISA resource name out"=w406:refnum<visa-resource-name>, "error out"=w407:errorcluster)  [unwired: 5 in]
            n150 = VISA Set I/O Buffer Size(VISA resource name=w406, mask (16)=w408, size (4096)=u32 24, error in (no error)=w407) -> (VISA resource name out=w402:refnum<visa-resource-name>, error out=w404:errorcluster)
            n151 = local write "VISA resource name out"(w406) -> ()
            n152 = disable-structure shown="Enabled" {
              disable-tunnel: w404 -> [w423 w424]
              disable-tunnel: [w422 w424] -> w403
              disable-tunnel: w402 -> [w421 _]
              disable-tunnel: w401 -> [w420 _]
              disable-tunnel: u32 24 ("size (4096)") -> [w419 _]
              frame Disabled {
                n153 = VISA Set I/O Buffer Size(VISA resource name=w421, mask (16)=w420, size (4096)=w419, error in (no error)=w423) -> (error out=w422:errorcluster)  [unwired: 1 out]
              }
              frame Enabled {
              }
            }
            n154 = Unbundle By Name(w403) -> ("status"=w409:bool)
            n155 = Not(x=w409) -> (.not. x?=w398:bool)
            n156 = Wait (ms)(milliseconds to wait=u32 50) -> ()  [unwired: 1 out]
            n157 = local write "STM _SeialConnected"(w398) -> ()
          }
          event "DISCONNECT": Value Change {
            n158 = event-data() -> ()  [unwired: 1 in, 6 out]
            n159 = local read "VISA resource name out"() -> (w428:refnum<visa-resource-name>)
            n160 = VISA Close(VISA resource name=w428, error in (no error)=w427) -> (error out=w426:errorcluster)
            n161 = Unbundle(w426) -> ("status"=w425:bool)  [unwired: 2 out]
            n162 = local write "STM _SeialConnected"(w425) -> ()
          }
          event "velocity_profileM1": Value Change {
            n163 = event-data() -> ()  [unwired: 1 in, 6 out]
            n164 = local read "STM _SeialConnected"() -> (w431:bool)
            n165 = case shown="True" w431 {
              tunnel: [w432 w453] -> w430
              tunnel: w429 -> [w432 w454]
              frame False {
              }
              frame True {
                w450 = "m" ("string")
                n166 = local read "Target_speed_M1"() -> (w434:i32)
                n167 = local read "ID_Motor1"() -> (w452:u8)
                n168 = Number To Decimal String(number=w452) -> (decimal integer string=w451:string)  [unwired: 1 in]
                n169 = Multiply(x=2.0, y=3.141592653589793) -> (x*y=w437:dbl)
                n170 = local read "VISA resource name out"() -> (w455:refnum<visa-resource-name>)
                n171 = Multiply(x=60.0, y=w434) -> (x*y=w440:dbl)
                n172 = Multiply(x=w437, y=140.0 ("x")) -> (x*y=w435:dbl)
                n173 = Divide(x=w440, y=w435) -> (x/y=w433:dbl)
                n174 = Negate(x=w433) -> (-x=w445:dbl)
                n175 = To Unsigned Long Integer(number=w445) -> (unsigned 32bit integer=w446:u32)
                n176 = Number To Boolean Array(number=w446) -> (Boolean array=w444:bool[])
                n177 = Boolean To (0,1)(Boolean=w444) -> (0, 1=w443:i16[])
                n178 = Number To Decimal String(number=w443) -> (decimal integer string=w442:string[])  [unwired: 1 in]
                n179 = Concatenate Strings(w451, w450, w450, "3" ("string"), "0" ("string"), "V" ("string"), w442) -> (w456:string)
                n180 = VISA Write(VISA resource name=w455, write buffer=w456, error in (no error)=w454) -> (error out=w453:errorcluster)  [unwired: 2 out]
              }
            }
          }
          event "position_profile_M1": Value Change {
            n181 = event-data() -> ()  [unwired: 1 in, 6 out]
            n182 = local read "STM _SeialConnected"() -> (w457:bool)
            n183 = case shown="False" w457 {
              tunnel: [w460 w474] -> w459
              tunnel: w458 -> [w460 w475]
              frame False {
              }
              frame True {
                w472 = "m" ("string")
                n184 = local read "ID_Motor1"() -> (w461:u8)
                n185 = local read "Target_Position_M1"() -> (w462:i32)
                n186 = Number To Decimal String(number=w461) -> (decimal integer string=w473:string)  [unwired: 1 in]
                n187 = local read "VISA resource name out"() -> (w463:refnum<visa-resource-name>)
                n188 = Negate(x=w462) -> (-x=w467:i32)
                n189 = To Unsigned Long Integer(number=w467) -> (unsigned 32bit integer=w468:u32)
                n190 = Number To Boolean Array(number=w468) -> (Boolean array=w466:bool[])
                n191 = Boolean To (0,1)(Boolean=w466) -> (0, 1=w465:i16[])
                n192 = Number To Decimal String(number=w465) -> (decimal integer string=w464:string[])  [unwired: 1 in]
                n193 = Concatenate Strings(w473, w472, w472, "1" ("string"), "0" ("string"), "P" ("string"), w464) -> (w476:string)
                n194 = VISA Write(VISA resource name=w463, write buffer=w476, error in (no error)=w475) -> (error out=w474:errorcluster)  [unwired: 2 out]
              }
            }
          }
          event "velocity_profileM2": Value Change {
            n195 = event-data() -> ()  [unwired: 1 in, 6 out]
            n196 = local read "STM _SeialConnected"() -> (w479:bool)
            n197 = case shown="True" w479 {
              tunnel: [w480 w502] -> w477
              tunnel: w478 -> [w480 w503]
              frame False {
              }
              frame True {
                w500 = "m" ("string")
                n198 = local read "ID_Motor2"() -> (w490:u8)
                n199 = local read "Target_speed_M2"() -> (w482:i32)
                n200 = Number To Decimal String(number=w490) -> (decimal integer string=w501:string)  [unwired: 1 in]
                n201 = local read "VISA resource name out"() -> (w491:refnum<visa-resource-name>)
                n202 = Multiply(x=2.0, y=3.141592653589793) -> (x*y=w485:dbl)
                n203 = Multiply(x=60.0, y=w482) -> (x*y=w488:dbl)
                n204 = Multiply(x=w485, y=140.0 ("x")) -> (x*y=w483:dbl)
                n205 = Divide(x=w488, y=w483) -> (x/y=w481:dbl)
                n206 = Negate(x=w481) -> (-x=w495:dbl)
                n207 = To Unsigned Long Integer(number=w495) -> (unsigned 32bit integer=w496:u32)
                n208 = Number To Boolean Array(number=w496) -> (Boolean array=w494:bool[])
                n209 = Boolean To (0,1)(Boolean=w494) -> (0, 1=w493:i16[])
                n210 = Number To Decimal String(number=w493) -> (decimal integer string=w492:string[])  [unwired: 1 in]
                n211 = Concatenate Strings(w501, w500, w500, "3" ("string"), "0" ("string"), "V" ("string"), w492) -> (w504:string)
                n212 = VISA Write(VISA resource name=w491, write buffer=w504, error in (no error)=w503) -> (error out=w502:errorcluster)  [unwired: 2 out]
              }
            }
          }
          event "position_profile_M2": Value Change {
            n213 = event-data() -> ()  [unwired: 1 in, 6 out]
            n214 = local read "STM _SeialConnected"() -> (w506:bool)
            n215 = case shown="True" w506 {
              tunnel: [w508 w522] -> w505
              tunnel: w507 -> [w508 w523]
              frame False {
              }
              frame True {
                w520 = "m" ("string")
                n216 = local read "ID_Motor2"() -> (w511:u8)
                n217 = local read "Target_Position_M2"() -> (w510:i32)
                n218 = Number To Decimal String(number=w511) -> (decimal integer string=w521:string)  [unwired: 1 in]
                n219 = Negate(x=w510) -> (-x=w515:i32)
                n220 = local read "VISA resource name out"() -> (w509:refnum<visa-resource-name>)
                n221 = To Unsigned Long Integer(number=w515) -> (unsigned 32bit integer=w516:u32)
                n222 = Number To Boolean Array(number=w516) -> (Boolean array=w514:bool[])
                n223 = Boolean To (0,1)(Boolean=w514) -> (0, 1=w513:i16[])
                n224 = Number To Decimal String(number=w513) -> (decimal integer string=w512:string[])  [unwired: 1 in]
                n225 = Concatenate Strings(w521, w520, w520, "1" ("string"), "0" ("string"), "P" ("string"), w512) -> (w524:string)
                n226 = VISA Write(VISA resource name=w509, write buffer=w524, error in (no error)=w523) -> (error out=w522:errorcluster)  [unwired: 2 out]
              }
            }
          }
          event "Homing_M1": Value Change {
            n227 = event-data() -> ()  [unwired: 1 in, 6 out]
            n228 = local read "STM _SeialConnected"() -> (w525:bool)
            n229 = case shown="True" w525 {
              tunnel: [w528 w550] -> w526
              tunnel: w527 -> [w528 w551]
              frame False {
              }
              frame True {
                w548 = "m" ("string")
                n230 = local read "ID_Motor1"() -> (w539:u8)
                n231 = local read "Target_speed_M1"() -> (w529:i32)
                n232 = Number To Decimal String(number=w539) -> (decimal integer string=w549:string)  [unwired: 1 in]
                n233 = Multiply(x=2.0, y=3.141592653589793) -> (x*y=w533:dbl)
                n234 = Multiply(x=60.0, y=w529) -> (x*y=w536:dbl)
                n235 = Multiply(x=w533, y=140.0 ("x")) -> (x*y=w531:dbl)
                n236 = local read "VISA resource name out"() -> (w538:refnum<visa-resource-name>)
                n237 = Divide(x=w536, y=w531) -> (x/y=w530:dbl)
                n238 = Negate(x=w530) -> (-x=w543:dbl)
                n239 = To Unsigned Long Integer(number=w543) -> (unsigned 32bit integer=w544:u32)
                n240 = Number To Boolean Array(number=w544) -> (Boolean array=w542:bool[])
                n241 = Boolean To (0,1)(Boolean=w542) -> (0, 1=w541:i16[])
                n242 = Number To Decimal String(number=w541) -> (decimal integer string=w540:string[])  [unwired: 1 in]
                n243 = Concatenate Strings(w549, w548, w548, "6" ("string"), "0" ("string"), "V" ("string"), w540) -> (w552:string)
                n244 = VISA Write(VISA resource name=w538, write buffer=w552, error in (no error)=w551) -> (error out=w550:errorcluster)  [unwired: 2 out]
              }
            }
          }
          event "Homing_M2": Value Change {
            n245 = event-data() -> ()  [unwired: 1 in, 6 out]
            n246 = local read "STM _SeialConnected"() -> (w553:bool)
            n247 = case shown="True" w553 {
              tunnel: [w556 w578] -> w554
              tunnel: w555 -> [w556 w579]
              frame False {
              }
              frame True {
                w576 = "m" ("string")
                n248 = local read "ID_Motor2"() -> (w567:u8)
                n249 = local read "Target_speed_M2"() -> (w557:i32)
                n250 = Number To Decimal String(number=w567) -> (decimal integer string=w577:string)  [unwired: 1 in]
                n251 = Multiply(x=2.0, y=3.141592653589793) -> (x*y=w561:dbl)
                n252 = local read "VISA resource name out"() -> (w566:refnum<visa-resource-name>)
                n253 = Multiply(x=60.0, y=w557) -> (x*y=w564:dbl)
                n254 = Multiply(x=w561, y=140.0 ("x")) -> (x*y=w559:dbl)
                n255 = Divide(x=w564, y=w559) -> (x/y=w558:dbl)
                n256 = Negate(x=w558) -> (-x=w571:dbl)
                n257 = To Unsigned Long Integer(number=w571) -> (unsigned 32bit integer=w572:u32)
                n258 = Number To Boolean Array(number=w572) -> (Boolean array=w570:bool[])
                n259 = Boolean To (0,1)(Boolean=w570) -> (0, 1=w569:i16[])
                n260 = Number To Decimal String(number=w569) -> (decimal integer string=w568:string[])  [unwired: 1 in]
                n261 = Concatenate Strings(w577, w576, w576, "6" ("string"), "0" ("string"), "V" ("string"), w568) -> (w580:string)
                n262 = VISA Write(VISA resource name=w566, write buffer=w580, error in (no error)=w579) -> (error out=w578:errorcluster)  [unwired: 2 out]
              }
            }
          }
        }
      }
      frame Error {
        (unwired) FALSE ("exit all")
        n263 = local write "error out"(w581) -> ()
      }
    }
    n264 = local write "error out"(w16) -> ()
    n265 = local read "exit all"() -> (w15:bool)
  }
  n266 = while {
    tunnel: w1 -> [w583]
    stop <- w585 stop-if-true
    n267 = local read "STM _SeialConnected"() -> (w584:bool)
    n268 = case shown="True" w584 {
      tunnel: w583 -> [_ w590]
      frame False {
        n269 = Wait (ms)(milliseconds to wait=u32 10) -> ()  [unwired: 1 out]
      }
      frame True {
        n270 = local read "VISA resource name out"() -> (w589:refnum<visa-resource-name>)
        n271 = VISA Read(VISA resource name=w589, byte count=u32 24, error in (no error)=w590) -> (read buffer=w588:string, error out=w587:errorcluster)  [unwired: 2 out]
        "read buffer" <- w588
        n272 = disable-structure shown="Enabled" {
          disable-tunnel: w588 -> [_ w597]
          frame Disabled {
          }
          frame Enabled {
            n273 = Match Pattern(string=w597, regular expression="\\") -> (before substring=w595:string, after substring=w596:string)  [unwired: 1 in, 2 out]
            n274 = Initialize Array(w595, 0 ("dimension size")) -> (w599:string[])
            n275 = while {
              shift-right: [w608] -> _
              shift-left: w596 -> [w612]
              shift-right: [w609] -> w592
              shift-left: w599 -> [w610]
              stop <- w606 stop-if-true
              # "oppure diverso"
              n276 = Match Pattern(string=w612, regular expression="\\") -> (before substring=w602:string, after substring=w608:string)  [unwired: 1 in, 2 out]
              n277 = Equal?(x="#", y=w602) -> (x = y?=w605:bool)
              n278 = case shown="True" w605 {
                tunnel: [w613 "0" ("x")] -> w603
                tunnel: w602 -> [w613 _]
                frame False {
                }
                frame True {
                }
              }
              n279 = Build Array (concatenate)(w610, w603) -> (w609:string[])
              n280 = Equal?(x=w608, y="" ("regular expression")) -> (x = y?=w606:bool)
            }
            n281 = Index Array(array=w592, index=23) -> (element=w593:string)
            n282 = case shown="\"L\", Default" w593 {
              tunnel: w592 -> [w601 _]
              frame "L", Default {
                n283 = Index Array(array=w601) -> ()  [unwired: 24 in, 24 out]
              }
              frame "H" {
              }
            }
          }
        }
        n284 = local write "error out"(w587) -> ()
      }
    }
    n285 = local read "exit all"() -> (w585:bool)
  }
  "error out" <- w4
